vi "Read From Spreadsheet File (I64).vi"(4 "delimiter (\\t)":string="\t", 6 "transpose (no:F)":bool, 7 "format (%d)":string="%d", 8 "max characters/row  (no limit:0)":i32, 9 "start of read offset (chars.:0)":i32, 10 "number of rows (all:-1)":i32=-1, 11 "file path (dialog if empty)":path) -> (0 "EOF?":bool, 1 "mark after read (chars.)":i32, 2 "first row":i64[](array[numeric]), 3 "all rows":i64[][](array[numeric]), 5 "new file path (Not A Path if cancelled)":path)   [LabVIEW 2020]
doc: "LabVIEW no longer supports this VI. Use the Read Delimited Spreadsheet VI instead.\n\nReads a specified number of lines or rows from a numeric text file beginning at a specified character offset and converts the data to a 2D, double-precision array of numbers, strings, or integers. You must manually select the polymorphic instance you want to use.\n\nYou optionally can transpose the array. The VI opens the file before reading from it and closes it afterwards. You can use this VI to read a spreadsheet file saved in text format. This VI calls the Spreadsheet String to Array function to convert the data."
panel:
  in  "type (empty)":i64[][](array[numeric])
  # "row\ncolumn"
  # "This VI is deprecated. Use the following VI instead:\n\nvi.lib\\Utility\\file.llb\\Read Delimited Spreadsheet.vi"
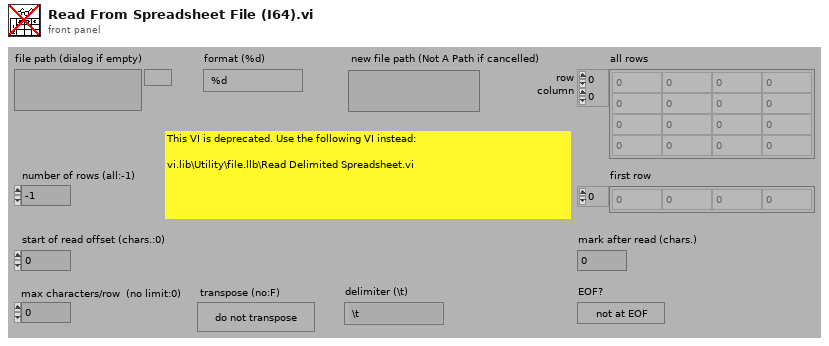
[diagram p1: front panel]
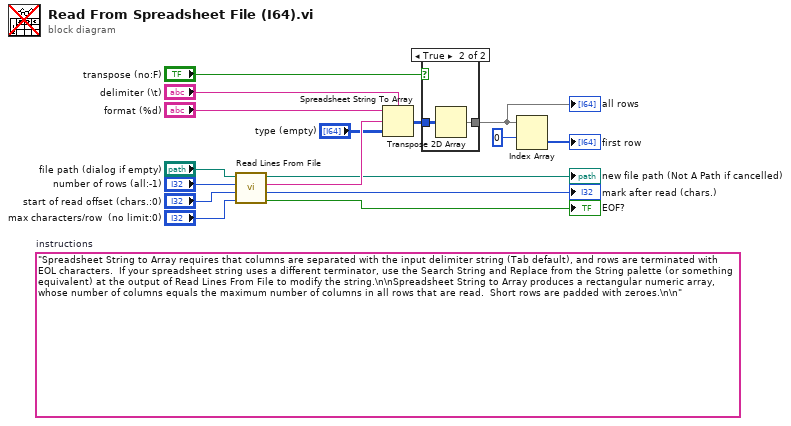
[diagram p0: block diagram]
diagram:
  (unwired) "Spreadsheet String to Array requires that columns are separated with the input delimiter string (Tab default), and rows are terminated with EOL characters.  If your spreadsheet string uses a different terminator, use the Search String and Replace from the String palette (or something equivalent) at the output of Read Lines From File to modify the string.\n\nSpreadsheet String to Array produces a rectangular numeric array, whose number of columns equals the maximum number of columns in all rows that are read.  Short rows are padded with zeroes.\n\n"  # instructions
  n1 = call "Read Lines From File.vi"("file path (dialog if empty)"="file path (dialog if empty)", "number of lines (all:-1)"="number of rows (all:-1)", "start of read offset (chars.:0)"="start of read offset (chars.:0)", "[max characters per line]  (no limit:0)"="max characters/row  (no limit:0)") -> ("new file path (Not A Path if cancelled)"=→"new file path (Not A Path if cancelled)":path, "line string"=w12:string, "mark after read (chars.)"=→"mark after read (chars.)":i32, "EOF?"=→"EOF?":bool)  [unwired: 2 in]
  n2 = Spreadsheet String To Array(delimiter (Tab)="delimiter (\\t)", format string="format (%d)", spreadsheet string=w12, array type (2D Dbl)="type (empty)") -> (array=w10:i64[][])
  n3 = case shown="True" "transpose (no:F)" {
    tunnel: [w17 w19] -> w7
    tunnel: w10 -> [w17 w18]
    frame False {
    }
    frame True {
      n4 = Transpose 2D Array(2D array=w18) -> (transposed array=w19:i64[][])
    }
  }
  "all rows" <- w7
  n5 = Index Array(array=w7, index (row)=0) -> (element=→"first row":i64[])  [unwired: 1 in]
